vi "VRM_sweepVsg_lockin.vi"(4 "Max Field for Triangle":dbl=1.05 min=-2.0 max=2.0 step=0.01, 5 "Offset":dbl min=-5.0 max=5.0 step=0.01, 6 "Ring":u16(ring) items=["Constant Field Sweep", "R - trangle wave"], 7 "Sweep rate (T/min)":dbl=0.02, 8 "Comments":string="Vbg=0.7V\n\nsweep Bx: 0T --> 2T, 0.02T/min\nsweep Vsg:  -60mV to 60mV, 100uV steps\n\nLockin\n0:18\n1: 19 0.5mV, phase=0\n2: 21\n3: 22\n4: 23\n5: 24\n\ndrive 19, 0.5mV 13.46Hz", 9 "ITX folder":string="7 - lockin_sweepB,Vsg", 10 "Measurement type":i32, 11 "Parameters":T1={"R1"=0.0, "R2"=1.9, "Phi1 (deg)"=0.0, "Phi2 (deg)"=0.0, "Theta1 (deg)"=90.0, "Theta2 (deg)"=90.0, "Step Size (T/deg/deg)"=1.9, "Stepping Parameter"=enum."R"} {"Theta2 (deg)" format="%#_13g"; "Theta1 (deg)" format="%#_13g"; "Phi2 (deg)" format="%#_13g"; "Phi1 (deg)" format="%#_13g"; "R2" format="%#_13g"; "R1" format="%#_13g"}) -> (0 "error out":errorcluster)   [LabVIEW 2013]
panel:
  in  "OK Button":bool
  in  "error in (no error)":errorcluster
  in  "stop":bool
  # "0=lockin\n1=IV"
  # "0: LOCKIN SWEEP VSG\n1: IV CURVES\nTheta: Azimuthal \nPhi: Polar (from Z down)\nThe ordering is the same as VRM."
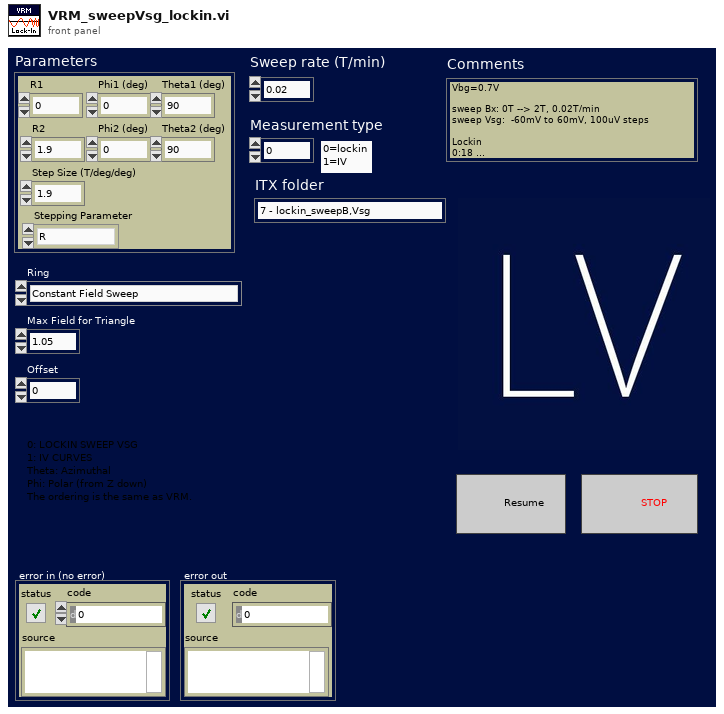
[diagram p1: front panel]
types:
  T1 = cluster{"R1":dbl, "R2":dbl, "Phi1 (deg)":dbl, "Phi2 (deg)":dbl, "Theta1 (deg)":dbl, "Theta2 (deg)":dbl, "Step Size (T/deg/deg)":dbl, "Stepping Parameter":enum16{"R", "Theta", "Phi"}}
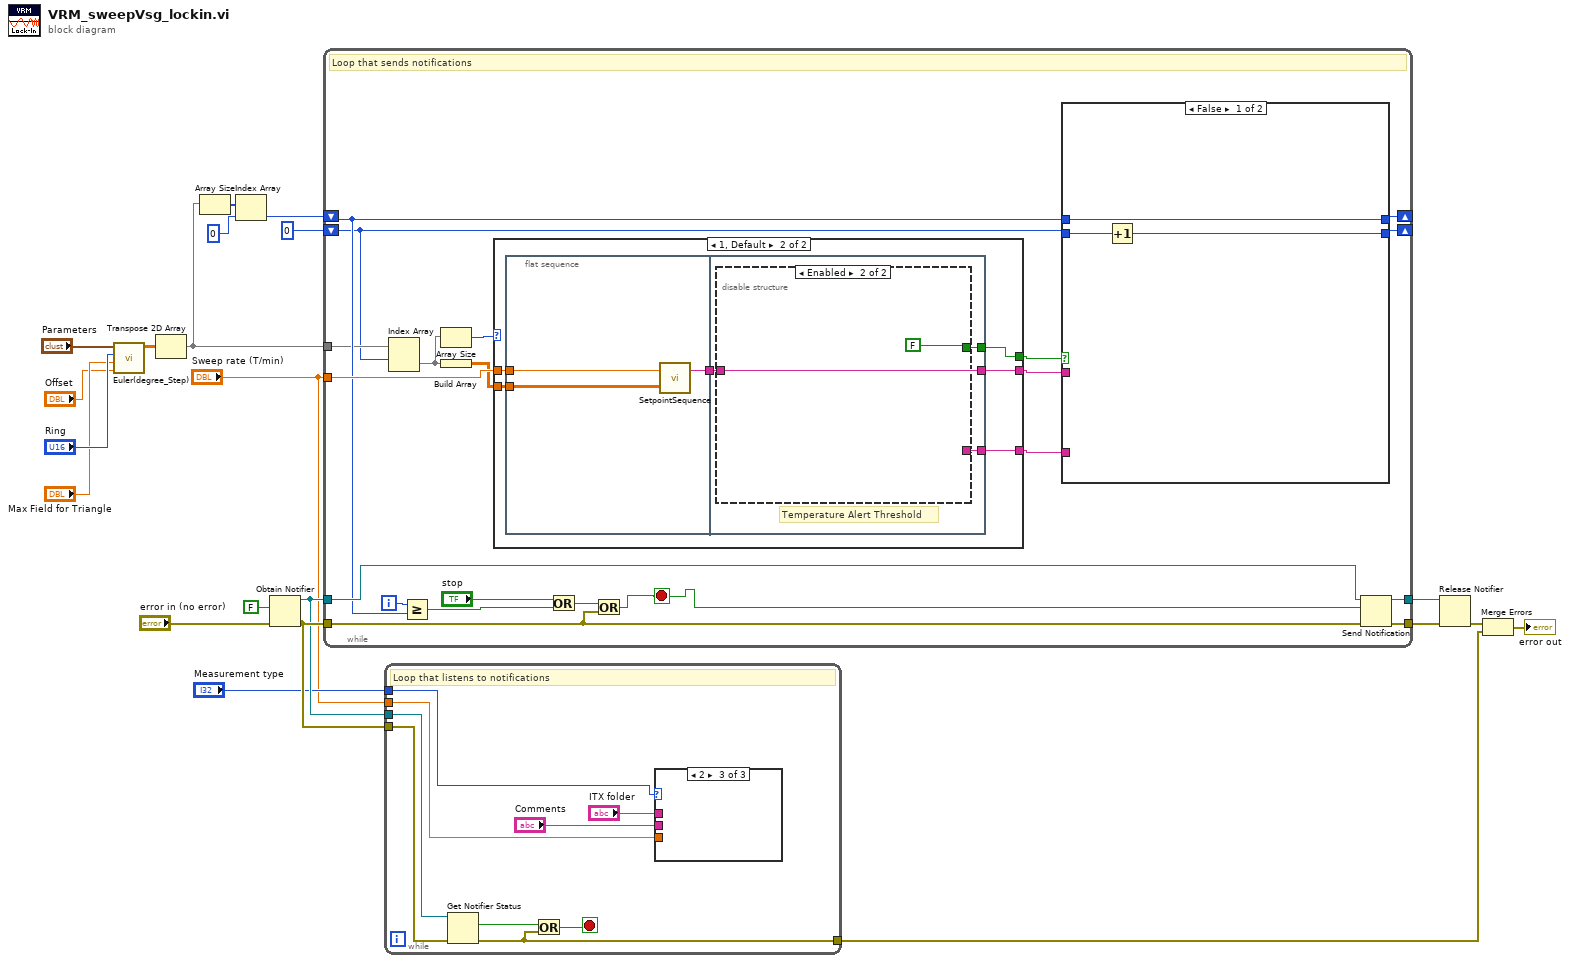
[diagram p0: block diagram]
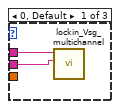
[diagram p2: hidden frame]
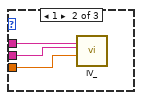
[diagram p3: hidden frame]
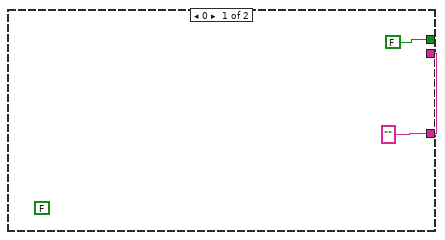
[diagram p4: hidden frame]
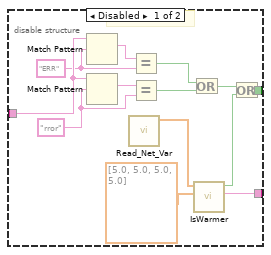
[diagram p5: hidden frame]
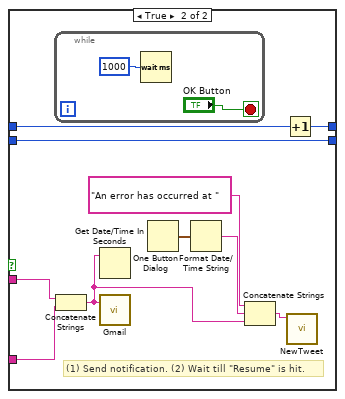
[diagram p6: hidden frame]
diagram:
  n1 = call "Euler(degree_Step).vi"("Offset"="Offset", "Max Field for Triangle"="Max Field for Triangle", "Ring"="Ring", "Cluster"="Parameters") -> ("Waveform Graph"=w18:dbl[][])  [unwired: 7 in]
  n2 = Transpose 2D Array(2D array=w18) -> (transposed array=w14:dbl[][])
  n3 = Array Size(array=w14) -> (size(s)=w16:i32[])
  n4 = Index Array(array=w16, index=0) -> (element=w15:i32)
  n5 = Obtain Notifier(notification data type=FALSE, error in (no error)="error in (no error)") -> (notifier out=w20:refnum<notifier>, error out=w21:errorcluster)  [unwired: 2 in, 1 out]
  n6 = while {
    tunnel: w20 -> [w39]
    tunnel: w21 -> [w33]
    tunnel: [w42] -> w1
    tunnel: [w41] -> w13
    tunnel: "Sweep rate (T/min)" -> [w40]
    tunnel: w14 -> [w26]
    shift-right: [w28] -> _
    shift-left: w15 -> [w29]
    shift-right: [w27] -> _
    shift-left: 0 -> [w24]
    i -> [w37]
    stop <- w22 stop-if-true
    # "Loop that sends notifications"
    n7 = Index Array(array=w26, index (row)=w24) -> (element=w25:dbl[])  [unwired: 1 in]
    n8 = Greater Or Equal?(x=w37, y=w29) -> (x >= y?=w38:bool)
    n9 = Array Size(array=w25) -> (size(s)=w32:i32)
    n10 = Build Array(w25) -> (w35:dbl[][])
    n11 = case shown="1, Default" w32 {
      tunnel: w40 -> [_ w50]
      tunnel: w35 -> [_ w49]
      tunnel: [w43 w48] -> w31
      tunnel: [FALSE w47] -> w30
      tunnel: [w43 w46] -> w23
      frame 0 {
        (unwired) FALSE
        w43 = "" ("Status")
      }
      frame 1, Default {
        n12 = flat-sequence {
          tunnel: w50 -> [w53]
          tunnel: w49 -> [w52]
          tunnel: [w51] -> w45
          tunnel: w45 -> [w56]
          tunnel: [w55] -> w47
          tunnel: [w56] -> w48
          tunnel: [w54] -> w46
          frame #0 {
            n13 = call "SetpointSequence.vi"("appended array"=w52, "Sweep rate (T/min)"=w53) -> ("Status"=w51:string)  [unwired: 1 in]
          }
          frame #1 {
            # "Temperature Alert Threshold"
            n14 = disable-structure shown="Enabled" {
              disable-tunnel: w56 -> [w69 _]
              disable-tunnel: [w68 FALSE] -> w55
              disable-tunnel: [w67 _] -> w54
              frame Disabled {
                w63 = "rror" ("regular expression")
                w65 = "ERR" ("regular expression")
                # "Error From VRM"
                n15 = Match Pattern(string=w69, regular expression=w65) -> (match substring=w66:string)  [unwired: 1 in, 3 out]
                n16 = Match Pattern(string=w69, regular expression=w63) -> (match substring=w64:string)  [unwired: 1 in, 3 out]
                n17 = call "Read_Net_Var.vi"() -> ("Array"=w57:dbl[])  [unwired: 11 in]
                n18 = Equal?(x=w66, y=w65) -> (x = y?=w62:bool)
                n19 = Equal?(x=w64, y=w63) -> (x = y?=w61:bool)
                n20 = Or(x=w62, y=w61) -> (x .or. y?=w59:bool)
                n21 = call "IsWarmer.vi"("Alert Threshold"=dbl[] [5.0, 5.0, 5.0, 5.0], "Temperature In"=w57) -> ("String"=w67:string, "Temperature is above threshold"=w58:bool)  [unwired: 8 in]
                n22 = Or(x=w59, y=w58) -> (x .or. y?=w68:bool)
              }
              frame Enabled {
              }
            }
          }
        }
      }
    }
    n23 = Or(x="stop", y=w38) -> (x .or. y?=w34:bool)
    n24 = Or(x=w34, y=w33) -> (x .or. y?=w22:bool)
    n25 = case shown="False" w30 {
      tunnel: [w73 w81] -> w27
      tunnel: [w72 w83] -> w28
      tunnel: w31 -> [_ w76]
      tunnel: w29 -> [w72 w82]
      tunnel: w24 -> [w71 w81]
      tunnel: w23 -> [_ w77]
      frame False {
        n26 = Increment(x=w71) -> (x+1=w73:i32)
      }
      frame True {
        # "(1) Send notification. (2) Wait till \"Resume\" is hit."
        n27 = while {
          stop <- "OK Button" stop-if-true
          n28 = Wait (ms)(milliseconds to wait=u32 1000) -> ()  [unwired: 1 out]
        }
        n29 = Concatenate Strings(w76, w77) -> (w75:string)
        n30 = One Button Dialog(message=w75) -> ()  [unwired: 1 in, 1 out]
        n31 = call "Gmail.vi"("Message Main Body"=w75) -> ()  [unwired: 3 in]
        n32 = Get Date/Time In Seconds() -> (seconds since 1Jan1904=w80:timestamp)
        n33 = Format Date/Time String(seconds (now)=w80) -> (date/time string=w79:string)  [unwired: 2 in]
        n34 = Concatenate Strings("An error has occurred at " ("string"), w79, w75) -> (w78:string)
        n35 = Increment(x=w82) -> (x+1=w83:i32)
        n36 = call "NewTweet.vi"("Message Main Body"=w78) -> ()  [unwired: 11 in]
      }
    }
    n37 = Send Notification(notification=w22, notifier=w39, error in (no error)=w33) -> (notifier out=w42:refnum<notifier>, error out=w41:errorcluster)
  }
  n38 = while {
    tunnel: w21 -> [w93]
    tunnel: w20 -> [w94]
    tunnel: "Measurement type" -> [w92]
    tunnel: [w88] -> w7
    tunnel: "Sweep rate (T/min)" -> [w91]
    stop <- w86 stop-if-true
    # "Loop that listens to notifications"
    n39 = Get Notifier Status(notifier=w94, error in (no error)=w93) -> (current notification=w87:bool, error out=w88:errorcluster)  [unwired: 3 out]
    n40 = Or(x=w87, y=w88) -> (x .or. y?=w86:bool)
    n41 = case shown="2" w92 {
      tunnel: "ITX folder" -> [w96 w99 _]
      tunnel: "Comments" -> [w95 w98 _]
      tunnel: w91 -> [_ w97 _]
      frame 0, Default {
        n42 = call "lockin_Vsg_multichannel.vi"("Comments"=w95, "ITX folder"=w96) -> ()  [unwired: 10 in]
      }
      frame 1 {
        n43 = call "IV_.vi"("B rate"=w97, "Notes"=w98, "Experiment folder name"=w99) -> ()  [unwired: 9 in]
      }
      frame 2 {
      }
    }
  }
  n44 = Release Notifier(notifier=w1, error in (no error)=w13) -> (error out=w6:errorcluster)  [unwired: 1 in, 2 out]
  n45 = Merge Errors(w6, w7) -> (→"error out":errorcluster)
